vi "Dashboard Main.vi"() -> ()   [LabVIEW 2013]
uses:
  <vilib>/event_ctls.llb/eventvkey.ctl
  <vilib>/Rock Robotics/WPI/Dashboard/WPI_DashboardLogging Global.vi
  <vilib>/Utility/config.llb/Write Key (String).vi
  <vilib>/Utility/config.llb/Write Key (I32).vi
  <vilib>/Utility/config.llb/NI_LVConfig.lvlib
panel:
  out "Camera Image":T1(plugin-control)
  out "LED 1":bool
  out "Image Message":string="Timeout in Camera Communications"
  in  "Rec Mode":enum32{"Stop", "Record", "Playback"}(radio)
  in  "Dashboard Tab":T2(tab)
  out "Shooter":bool
  in  "Camera Settings":T3={"Frame Rate"=30, "Compression"=30, "Size"=1} {"Frame Rate" scale=1.0..30.0; "Size" items=["640x480", "320x240", "160x120"]}
  out "MotorSliders R":cluster{"MotorSlide1":dbl, "MotorSlide2":dbl} {"MotorSlide2" scale=-1.0..1.0 scale format="%#_2e"; "MotorSlide1" scale=-1.0..1.0 scale format="%#_2e"}
  out "MotorChart R":cluster{"Numeric":dbl, "Numeric":dbl}(graph)
  out "MotorSliders L":T4 {"MotorSlide4 2" scale=0.0..14.0 scale format="%#_2e"; "MotorSlide2" scale=-1.0..1.0 scale format="%#_2e"; "MotorSlide1" scale=-1.0..1.0 scale format="%#_2e"}
  out "MotorChart L":T5(graph)
  out "JS1 Z":dbl(slide) scale=-1.0..1.0 scale format="%#_2e"
  out "Joystick 1":cluster{"X":dbl, "Y":dbl}[](graph)
  out "JS Buttons 1":T6
  out "JS2 Z":dbl(slide) scale=-1.0..1.0 scale format="%#_2e"
  out "Joystick 2":cluster{"X":dbl, "Y":dbl}[](graph)
  out "JS Buttons 2":T6
  out "Mode":T7(ring)=enum."Auto Disabled"
  out "Camera IP":string
  in  "DB Camera Config":bool
  out "fps":dbl format="%#.1g"
  out "Mbps":dbl format="%#.1g"
  out "Mbps 2":bool
  out "You're\nGood\nHomie":bool
  out "Distance Meter":dbl(knob) scale=36.0..60.0
  in  "Slider 1":dbl(slide) scale=0.0..100.0
  in  "Checkbox 2":bool
  in  "Checkbox 1":bool
  in  "Test Slider":dbl(slide) scale=0.0..100.0 scale format="%#_3g"
  in  "On/Off":bool caption="Solenoid"
  in  "Test Name":u16(ring) items=["Select the test to run...", "Example Test", "-------------------------------", "List of tests is built in robot code.", "Replace with your own automated tests."]
  in  "Test Tree":string(tree)
  in  "Motor":cluster{"Value":dbl, "Enable":bool} {"Value" scale=-1.0..1.0 scale format="%#_3g"}
  out "Progress":T8 {"Test Progress" scale=0.0..100.0}
  in  "Rev/Fwd":cluster{"Forward":bool, "Reverse":bool}
  in  "Test Ring":u16(ring) items=["Auto", "Fixed indoor", "Fixed outdoor 1", "Fixed outdoor 2", "Fixed fluorescent 1", "Fixed fluorescent 2", "Hold current"]
  in  "Listbox":i32(listbox)
  out "Tree":string(tree)
  in  "Enable":bool
  # "Left"
  # "Front"
  # "Right"
  # "Battery"
  # "Customize by placing controls and indicators here and name to\nmatch Dashboard Variables on robot."
  # "This tab is a great place for autonomous settings and validation.\nCustomize by placing controls and indicators here and name to\nmatch Dashboard Variables on robot."
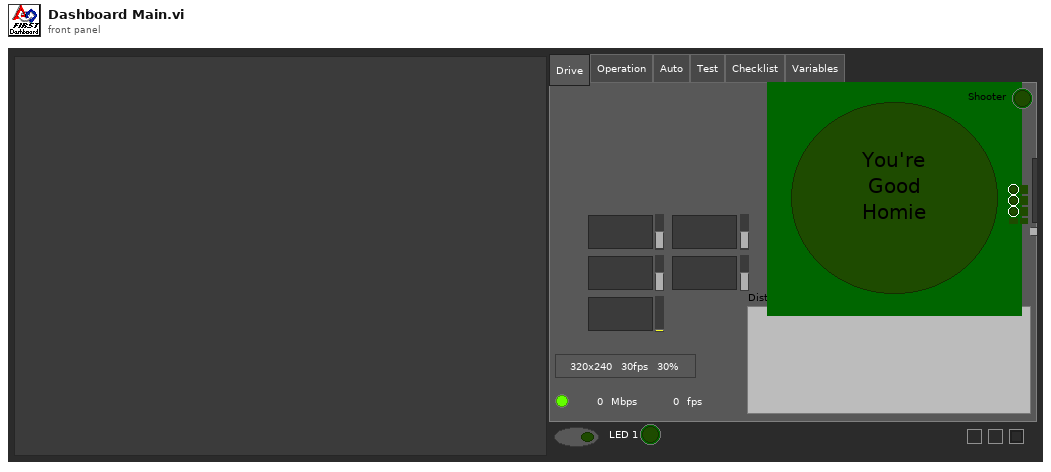
[diagram p1: front panel]
types:
  T1 = typedef "IMAQ Image.ctl" = refnum<image>
  T2 = enum32{"Drive", "Operation", "Auto", "Test", "Checklist", "Variables"}
  T3 = cluster{"Frame Rate":i32, "Compression":i32, "Size":u16}
  T4 = cluster{"MotorSlide1":dbl, "MotorSlide2":dbl, "MotorSlide4 2":dbl}
  T5 = cluster{"Numeric":dbl, "Numeric":dbl, "Battery":sgl}
  T6 = cluster{bool, bool, bool, bool, bool, bool, bool, bool, bool, bool, bool, bool}
  T7 = enum8{"Tele-Op Disabled", "Tele-Op Enabled", "Auto Disabled", "Auto Enabled", "Test Disabled", "Test Enabled", ""}
  T8 = cluster{"Test Progress":u8, "Test Progress Text":string}
  T9 = typedef "Image Type" = u32
  T10 = cluster{"X":bool, "A":bool, "B":bool, "Y":bool, "LB":bool, "RB":bool, "LT":bool, "RT":bool, "Back":bool, "Start":bool, "LC":bool, "RC":bool}
  T11 = cluster{"Pos. X":i32, "Pos. Y":i32, "Radius":i32, "Core Area":i32}[]
  T12 = cluster{"Pos. X":i32, "Pos. Y":i32, "Radius":i32, "Core Area":i32}
  T13 = typedef "NI_LVConfig.lvlib/Config Data RefNum.ctl" = refnum<k1>
  T14 = cluster{"Digital Inputs":bool[], "Digital Outputs":bool[]}
  T15 = cluster{"Competition mode":bool, "Robot Link":bool, "Autonomous":bool, "Enabled":bool, "E-Stop":bool, "Simulated":bool, "TestMode":bool, "Docked Window":bool}
  T16 = cluster{"Boolean Array[0]":bool, "Boolean Array[1]":bool, "Boolean Array[2]":bool, "Boolean Array[3]":bool, "Boolean Array[4]":bool, "Boolean Array[5]":bool, "Boolean Array[6]":bool, "Boolean Array[7]":bool, "Boolean Array[8]":bool, "Boolean Array[9]":bool, "Boolean Array[10]":bool, "Boolean Array[11]":bool}
  T17 = typedef "eventvkey.ctl" = enum16{"ASCII", "Enter", "Return", "Shift", "Ctrl", "Alt", "Cmd", "Opt", "Caps", "NumLock", "Clear", "Break", "Up", "Down", "Left", "Right", "Insert", "Delete", "Home", "End", "PageUp", "PageDown", "Escape", "Help", "Pause", "ScrollLock", "F1", "F2", "F3", "F4", "F5", "F6", "F7", "F8", "F9", "F10", "F11", "F12", "F13", "F14", "F15", "F16", "F17", "F18", "F19", "F20", "F21", "F22", "F23", "F24", "Play", "VolumeUp", "VolumeDown", "Mute", "Two Byte Char"}
  T18 = cluster{"Image Size":bool, "Image Type":bool, "Pixel Value":bool, "ROI Information":bool, "Zoom Factor":bool}
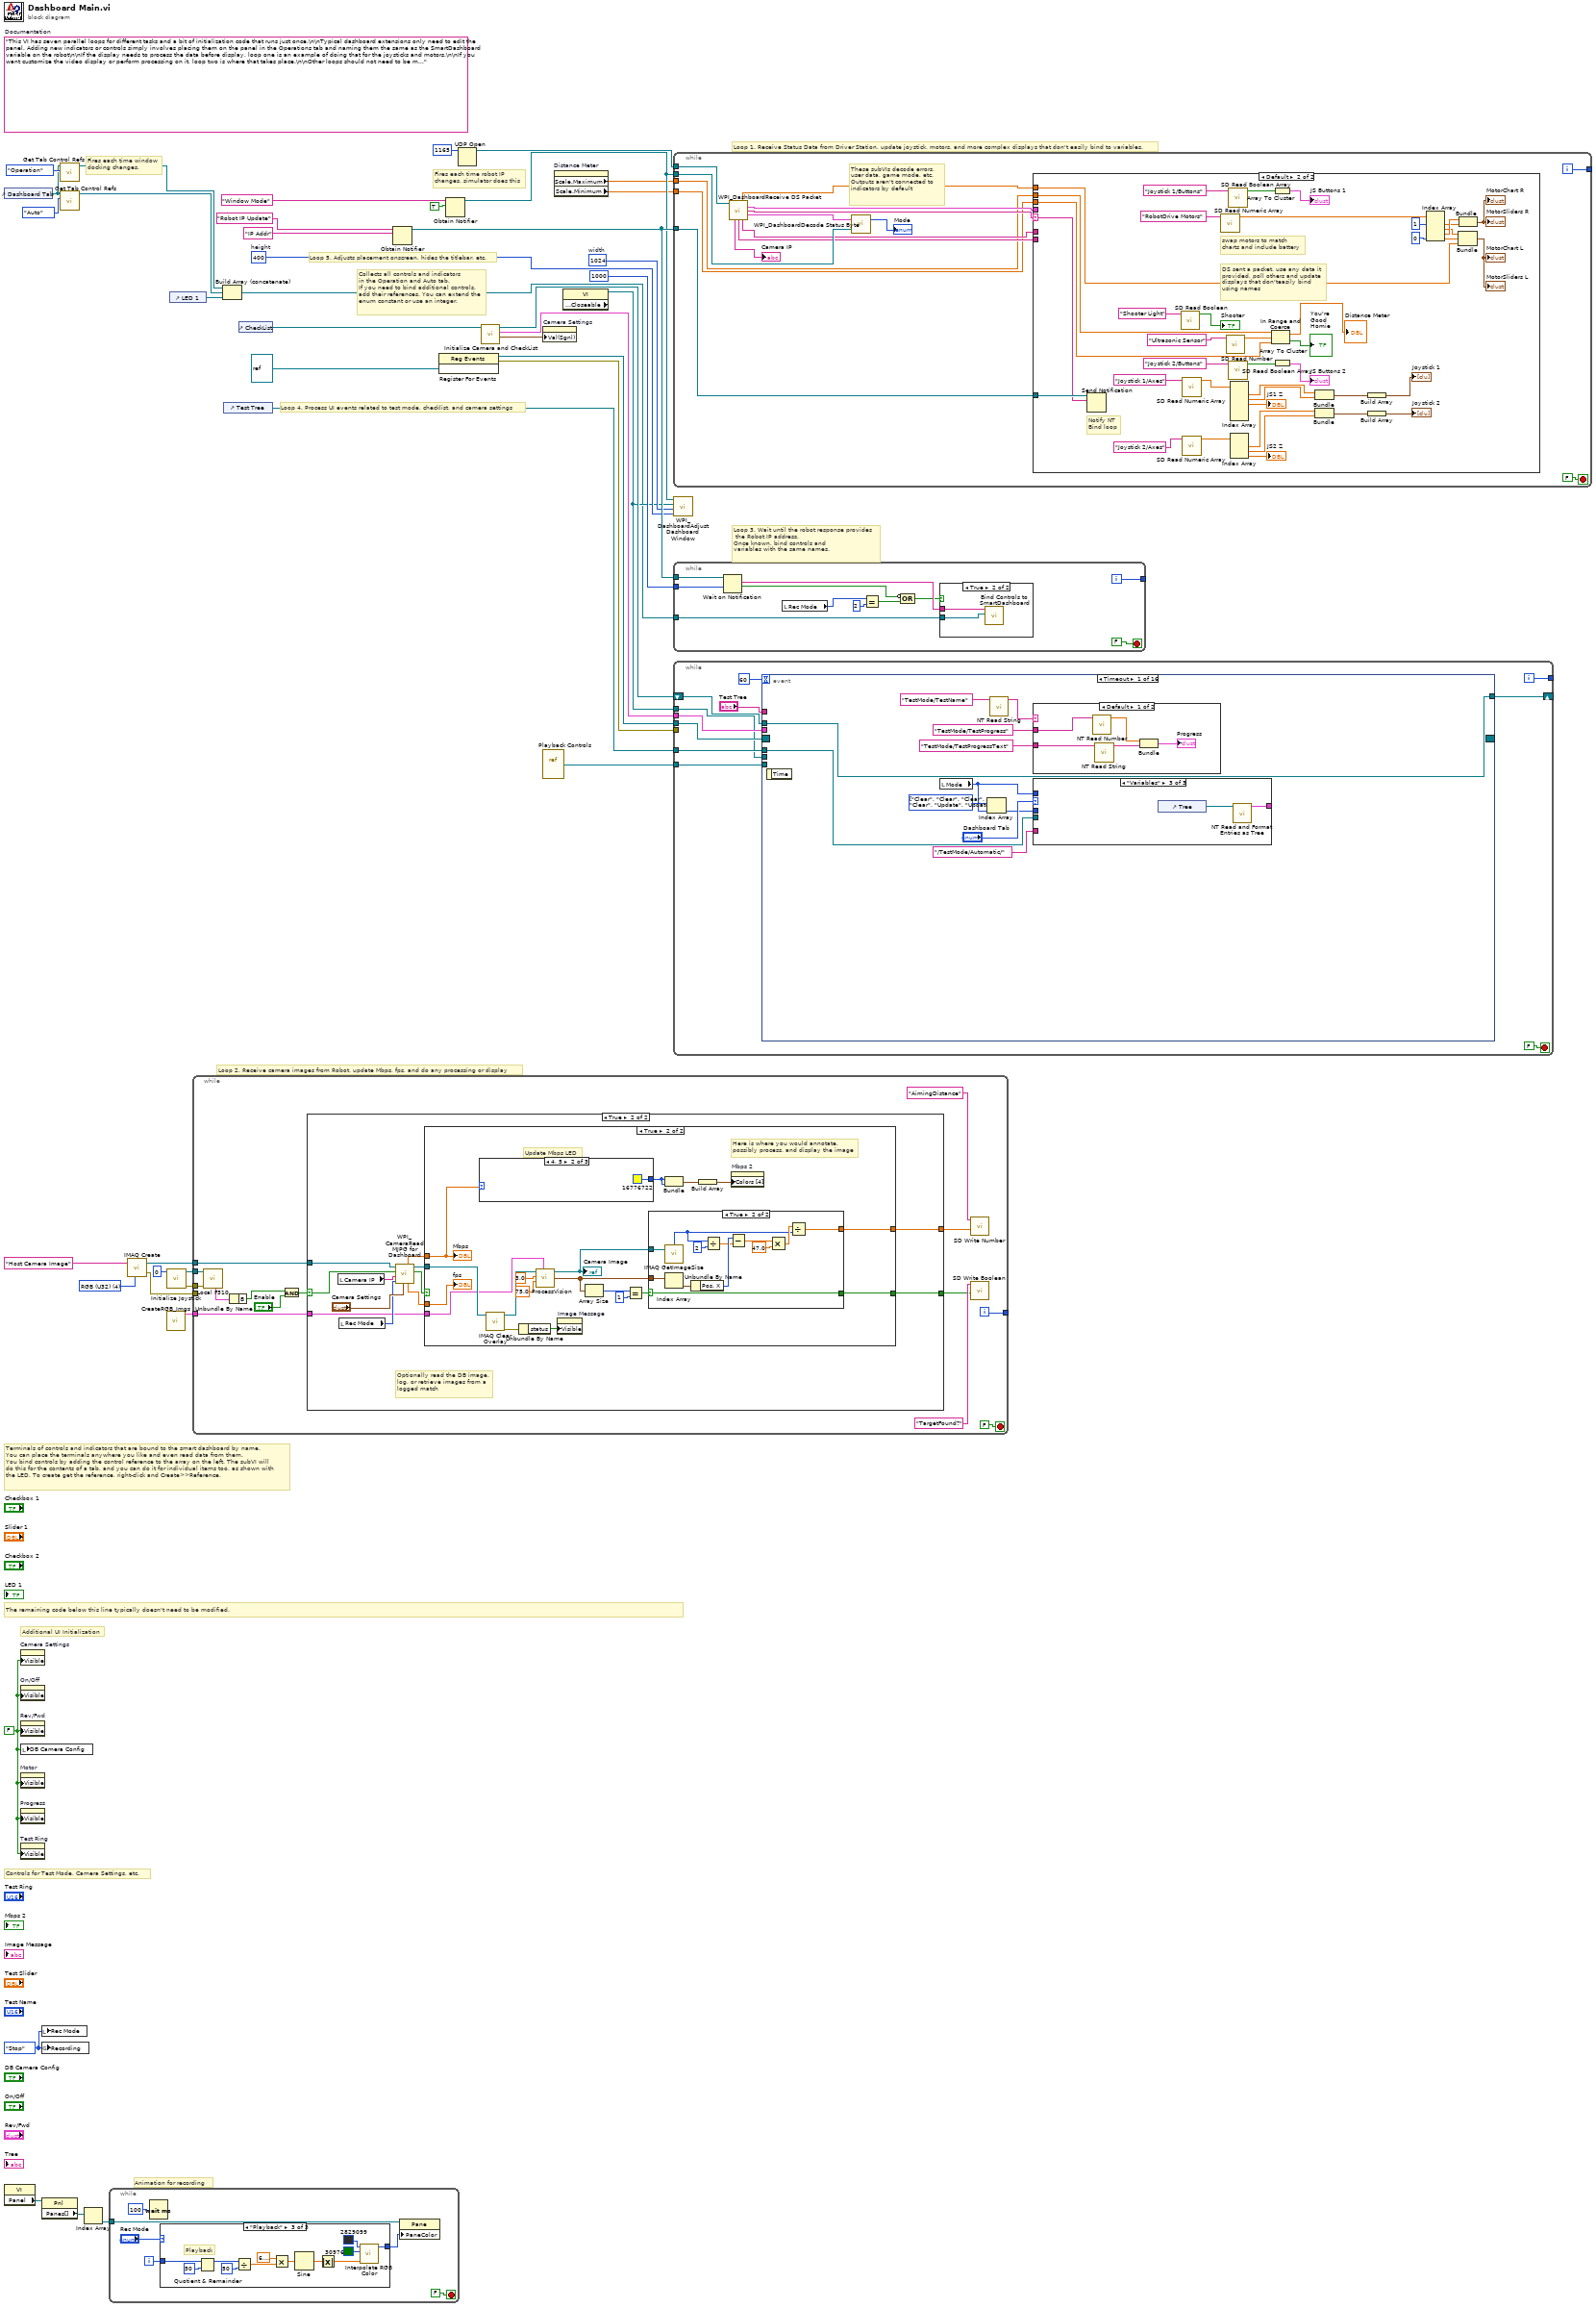
[diagram p0: block diagram]
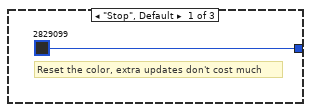
[diagram p2: hidden frame]
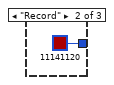
[diagram p3: hidden frame]
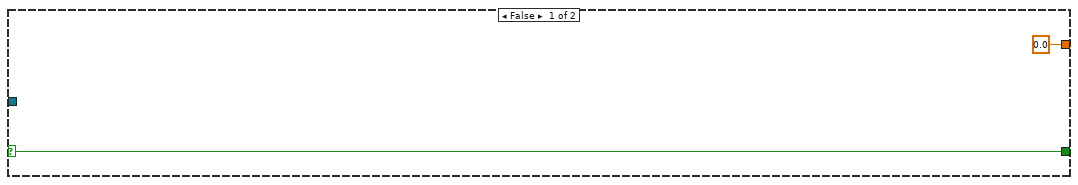
[diagram p5: hidden frame]
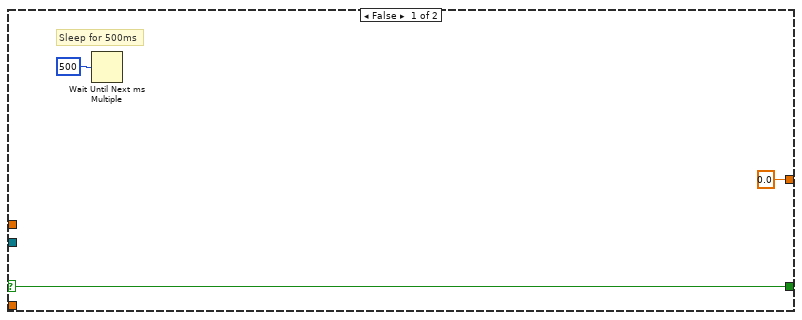
[diagram p6: hidden frame]
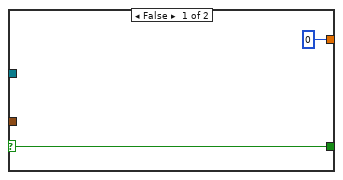
[diagram p7: hidden frame]
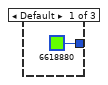
[diagram p8: hidden frame]
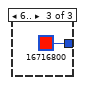
[diagram p9: hidden frame]
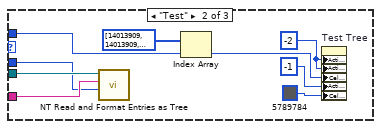
[diagram p11: hidden frame]
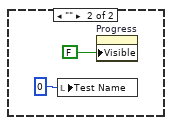
[diagram p12: hidden frame]
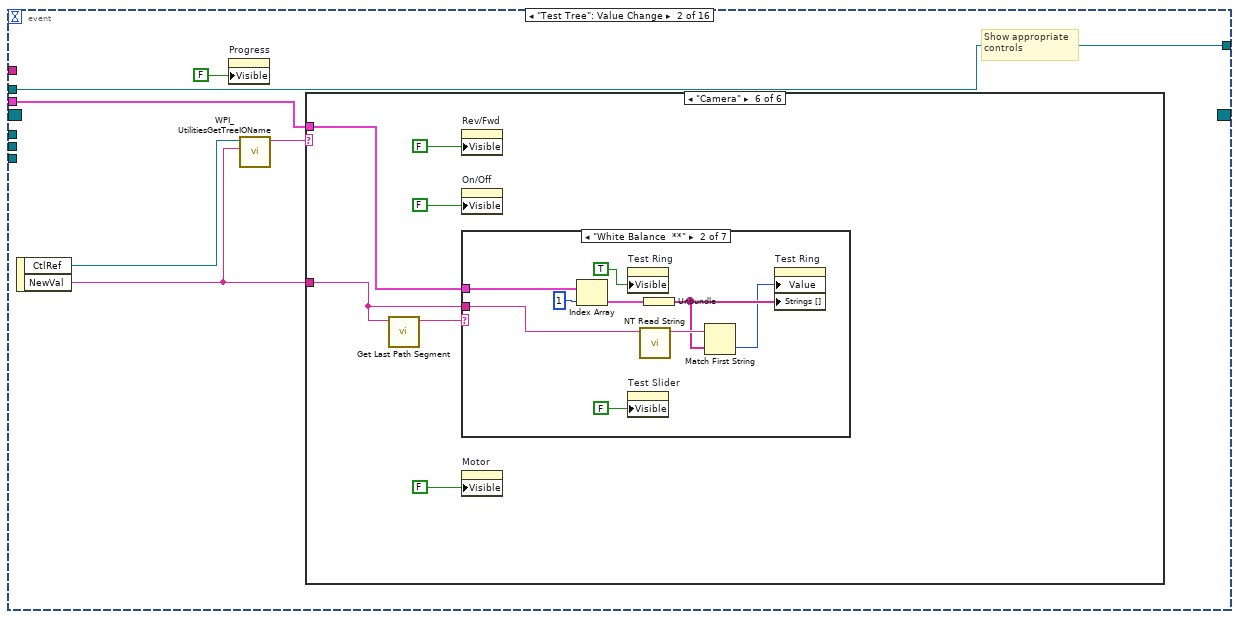
[diagram p13: hidden frame]
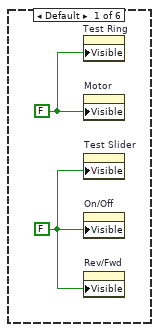
[diagram p14: hidden frame]
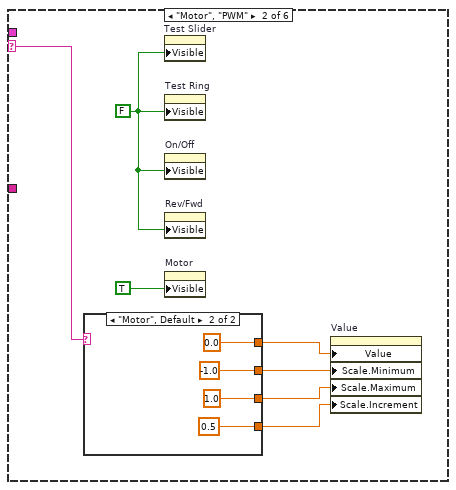
[diagram p15: hidden frame]
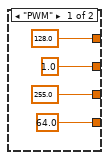
[diagram p16: hidden frame]
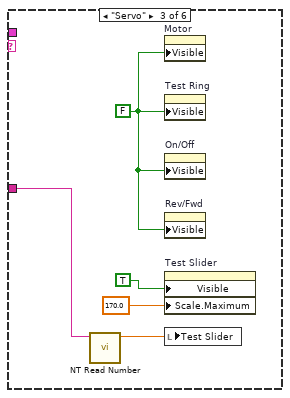
[diagram p17: hidden frame]
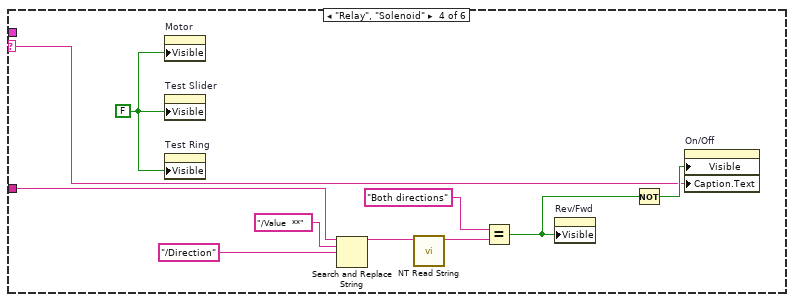
[diagram p18: hidden frame]
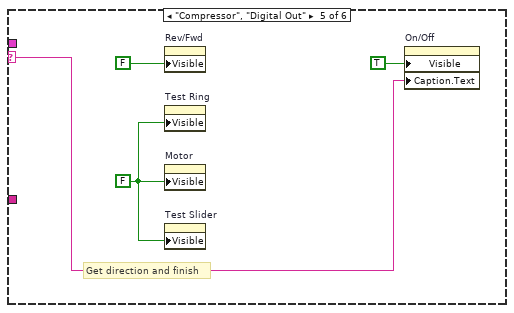
[diagram p19: hidden frame]
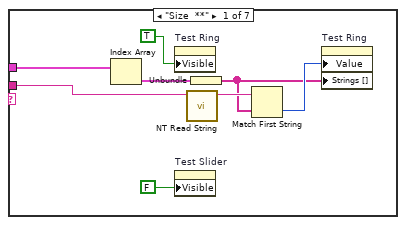
[diagram p20: hidden frame]
diagram:
  w14 = enum32{"Stop", "Record", "Playback"}."Stop" ("Rec Mode")
  w17 = 400  # height
  w18 = 1024  # width
  w31 = FALSE ("Visible")
  (unwired) "This VI has seven parallel loops for different tasks and a bit of initialization code that runs just once.\n\nTypical dashboard extensions only need to edit the panel. Adding new indicators or controls simply involves placing them on the panel in the Operations tab and naming them the same as the SmartDashboard variable on the robot\n\nIf the display needs to process the data before display, loop one is an example of doing that for the joysticks and motors.\n\nIf you want customize the video display or perform processing on it, loop two is where that takes place.\n\nOther loops should not need to be modified. They are pretty standard, and document the task they perform."  # Documentation
  w41 = T9 4 items=["Grayscale (U8)", "Grayscale (I16)", "Grayscale (SGL)", "Complex (CSG)", "RGB (U32)", "HSL (U32)", "RGB (U64)"] ("Image Type")
  # "Controls for Test Mode, Camera Settings, etc."
  # "Additional UI Initialization"
  # "Animation for recording"
  # "Fires each time robot IP\nchanges, simulator does this"
  # "Fires each time window\ndocking changes."
  # "Collects all controls and indicators\nin the Operation and Auto tab.\nIf you need to bind additional controls,\nadd their references. You can extend the\nenum constant or use an integer."
  # "The remaining code below this line typically doesn't need to be modified."
  # "Loop 4. Process UI events related to test mode, checklist, and camera settings"
  # "Terminals of controls and indicators that are bound to the smart dashboard by name.\nYou can place the terminals anywhere you like and even read data from them.\nYou bind controls by adding the control reference to the array on the left. The subVI will\ndo this for the contents of a tab, and you can do it for individual items too, as shown with\nthe LED. To create get the reference, right-click and Create>>Reference."
  # "Loop 3. Wait until the robot response provides\n the Robot IP address.\nOnce known, bind controls and\nvariables with the same names."
  # "Loop 5. Adjusts placement onscreen, hides the titlebar, etc."
  # "Loop 1. Receive Status Data from Driver Station, update joystick, motors, and more complex displays that don't easily bind to variables."
  # "Loop 2. Receive camera images from Robot, update Mbps, fps, and do any processing or display"
  n1 = control-ref of="Dashboard Tab"() -> (w12:refnum<vi>)
  n2 = property class="VI"() -> ("Panel"=w25:refnum<vi>)  [unwired: 2 in, 2 out]
  n3 = property on="Camera Settings" class="Clust (strict)"("Visible"=w31) -> ()  [unwired: 2 in, 2 out]
  n4 = property on="On/Off" class="Bool (strict)"("Visible"=w31) -> ()  [unwired: 2 in, 2 out]
  n5 = property on="Rev/Fwd" class="Clust (strict)"("Visible"=w31) -> ()  [unwired: 2 in, 2 out]
  n6 = local write "DB Camera Config"(w31) -> ()
  n7 = property on="Motor" class="Clust (strict)"("Visible"=w31) -> ()  [unwired: 2 in, 2 out]
  n8 = property on="Progress" class="Clust (strict)"("Visible"=w31) -> ()  [unwired: 2 in, 2 out]
  n9 = property on="Test Ring" class="Ring (strict)"("Visible"=w31) -> ()  [unwired: 2 in, 2 out]
  n10 = local write "Rec Mode"(w14) -> ()
  n11 = global write "WPI_DashboardLogging Global.vi" "Recording"(w14) -> ()
  n12 = property class="Pnl"(reference=w25) -> ("Panes[]"=w26:refnum<vi>[])  [unwired: 1 in, 2 out]
  n13 = call <vilib>:"Get Tab Control Refs.vi"("Page Index"=T2."Operation" ("Dashboard Tab"), "TabControl in"=w12) -> ("ControlsOnPage"=w10:refnum<vi>[])  [unwired: 9 in]
  n14 = call <vilib>:"Get Tab Control Refs.vi"("Page Index"=T2."Auto" ("Dashboard Tab"), "TabControl in"=w12) -> ("ControlsOnPage"=w11:refnum<vi>[])  [unwired: 9 in]
  n15 = Index Array(array=w26) -> (element=w24:refnum<vi>)  [unwired: 1 in]
  n16 = while {
    tunnel: w24 -> [w45]
    i -> [w48]
    stop <- FALSE stop-if-true
    n17 = Wait (ms)(milliseconds to wait=u32 100) -> ()  [unwired: 1 out]
    n18 = case shown="\"Playback\"" "Rec Mode" {
      tunnel: w48 -> [_ _ w63]
      tunnel: [u32 2829099 ("Base Color") u32 11141120 ("Target Color") w52] -> w44
      frame "Stop", Default {
        # "Reset the color, extra updates don't cost much"
      }
      frame "Record" {
      }
      frame "Playback" {
        # "Playback"
        n19 = Quotient & Remainder(x=w63, y=u32 50 ("milliseconds to wait")) -> (x-y*floor(x/y)=w59:u32)  [unwired: 1 out]
        n20 = Divide(x=w59, y=u32 50 ("milliseconds to wait")) -> (x/y=w56:dbl)
        n21 = Multiply(x=6.283185307179586, y=w56) -> (x*y=w61:dbl)
        n22 = Sine(x=w61) -> (sin(x)=w60:dbl)
        n23 = Absolute Value(x=w60) -> (abs(x)=w53:dbl)
        n24 = call "Interpolate RGB Color.vi"("Proportion"=w53, "Target Color"=u32 30976, "Base Color"=u32 2829099) -> ("Result Color"=w52:u32)  [unwired: 8 in]
      }
    }
    n25 = property class="Pane"(reference=w45, "PaneColor"=w44) -> ()  [unwired: 1 in, 2 out]
  }
  n26 = call "IMAQ Create"("Image Name"="Host Camera Image", "Image Type"=w41) -> ("New Image"=w39:T1, "error out"=w38:errorcluster)  [unwired: 2 in, 1 out]
  n27 = call "CreateRGB_Imgs.vi"() -> ("RGB Cluster"=w4:cluster{"Red":T1, "Green":T1, "Blue":T1})  [unwired: 3 out]
  n28 = call <vilib>:"Initialize Joystick.vi"("device index"=0) -> ("error out"=w2:errorcluster, "device ID"=w1:refnum<k1>)  [unwired: 9 in]
  n29 = control-ref of="LED 1"() -> (w7:refnum<vi>)
  n30 = while {
    tunnel: w39 -> [w75]
    tunnel: w38 -> [_]
    tunnel: [w76] -> _
    tunnel: w4 -> [w73]
    tunnel: w2 -> [w72]
    tunnel: w1 -> [w71]
    i -> [w76]
    stop <- FALSE stop-if-true
    n31 = call "Local F310.vi"("error in (no error)"=w72, "device ID"=w71) -> ("Buttons"=w70:T10)  [unwired: 4 in, 5 out]
    n32 = Unbundle By Name(w70) -> ("B"=w69:bool)
    n33 = And(x=w69, y="Enable") -> (x .and. y?=w68:bool)
    n34 = case shown="True" w68 {
      selector: w68 -> [w79 w80]
      tunnel: w75 -> [_ w91]
      tunnel: w73 -> [_ w83]
      tunnel: [0.0 ("Pos. X") w82] -> w65
      tunnel: [w79 w81] -> w64
      frame False {
      }
      frame True {
        # "Optionally read the DB image,\nlog, or retrieve images from a\nlogged match"
        n35 = local read "Camera IP"() -> (w85:string)
        n36 = local read "Rec Mode"() -> (w84:enum32{"Stop", "Record", "Playback"})
        n37 = call <vilib>:"WPI_CameraRead MJPG for Dashboard.vi"("Camera Settings"="Camera Settings", "Rec Mode"=w84, "Camera IP"=w85, "Enable"=w80, "Refnum in"=w91) -> ("Active"=w89:bool, "Refnum out"=w90:T1, "FPS"=w88:dbl, "Bandwidth (Mbps)"=w87:dbl)  [unwired: 3 in]
        n38 = case shown="True" w89 {
          selector: w89 -> [w93 _]
          tunnel: w90 -> [_ w108]
          tunnel: w87 -> [_ w107]
          tunnel: w88 -> [_ w106]
          tunnel: w83 -> [_ w98]
          tunnel: [0.0 ("Pos. X") w96] -> w82
          tunnel: [w93 w95] -> w81
          frame False {
            # "Sleep for 500ms"
            n39 = Wait Until Next ms Multiple(millisecond multiple=u32 500) -> ()  [unwired: 1 out]
          }
          frame True {
            # "Here is where you would annotate,\npossibly process, and display the image"
            # "Update Mbps LED"
            n40 = case shown="4, 5" w107 {
              tunnel: [u32 6618880 ("Color Box") u32 16776722 ("Color Box") u32 16716800 ("Color Box")] -> w109
              frame Default {
              }
              frame 4, 5 {
              }
              frame 6.. {
              }
            }
            n41 = call "IMAQ Clear Overlay"("Image"=w108) -> ("error out"=w112:errorcluster, "Image Out"=w102:T1)  [unwired: 2 in, 7 out]
            n42 = Unbundle By Name(w112) -> ("status"=w113:bool)
            n43 = call "ProcessVision.vi"("Image Src"=w102, "Min Radius"=sgl 3.0, "Max Radius"=sgl 75.0, "RGB Cluster"=w98) -> ("Image Out"=w97:T1, "Circles Data"=w99:T11)  [unwired: 1 in, 1 out]
            "Camera Image" <- w97
            n44 = property on="Image Message" class="Str"("Visible"=w113) -> ()  [unwired: 2 in, 2 out]
            n45 = Array Size(array=w99) -> (size(s)=w105:i32)
            n46 = Equal?(x=w105, y=1) -> (x = y?=w103:bool)
            n47 = case shown="True" w103 {
              selector: w103 -> [w114 w127]
              tunnel: [0 ("Pos. X") w116] -> w96
              tunnel: [w114 w127] -> w95
              tunnel: w99 -> [_ w126]
              tunnel: w97 -> [_ w124]
              frame False {
              }
              frame True {
                n48 = call "IMAQ GetImageSize"("Image"=w124) -> ("X Resolution"=w117:i32)  [unwired: 3 in, 2 out]
                n49 = Index Array(array=w126) -> (element=w125:T12)  [unwired: 1 in]
                n50 = Unbundle By Name(w125) -> ("Pos. X"=w122:i32)
                n51 = Divide(x=w117, y=2) -> (x/y=w121:dbl)
                n52 = Subtract(x=w122, y=w121) -> (x-y=w120:dbl)
                n53 = Multiply(x=w120, y=47.0) -> (x*y=w118:dbl)
                n54 = Divide(x=w118, y=w117) -> (x/y=w116:dbl)
              }
            }
            n55 = Bundle("Color Box"=w109, "Color Box"=w109) -> (w111:cluster{"Color Box":u32, "Color Box":u32})  [unwired: 1 out]
            n56 = Build Array(w111) -> (w110:cluster{"Color Box":u32, "Color Box":u32}[])
            n57 = property on="Mbps 2" class="Bool (strict)"("Colors [4]"=w110) -> ()  [unwired: 2 in, 2 out]
            "Mbps" <- w107
            "fps" <- w106
          }
        }
      }
    }
    n58 = call <vilib>:"SD Write Number.vi"("Numeric"=w65, "Name"="AimingDistance") -> ()  [unwired: 8 in, 2 out]
    n59 = call <vilib>:"SD Write Boolean.vi"("Boolean"=w64, "Name"="TargetFound?") -> ()  [unwired: 8 in, 2 out]
  }
  n60 = Build Array (concatenate)(w10, w11, w7) -> (w9:refnum<vi>[])
  n61 = control-ref of="Test Tree"() -> (w27:refnum<vi>)
  n62 = control-ref of="CheckList"() -> (w15:refnum<vi>)
  n63 = Obtain Notifier(name (unnamed)="Robot IP Update", notification data type="IP Addr" ("name (unnamed)")) -> (notifier out=w35:refnum<notifier>)  [unwired: 2 in, 2 out]
  n64 = register-events(refnum<vi> refnum) -> (reference out=w22:refnum<event-registration>, error out=w21:errorcluster)  [unwired: 2 in]
  n65 = Obtain Notifier(name (unnamed)="Window Mode", notification data type=TRUE) -> (notifier out=w16:refnum<notifier>)  [unwired: 2 in, 2 out]
  n66 = UDP Open(11:u16 1165 ("port")) -> (port=w42:refnum<k16>)  [unwired: 2 in, 4 out]
  n67 = call "Initialize Camera and CheckList.vi"("ListBox in"=w15) -> ("Cluster"=w29:cluster{"value":i32, "value":i32, "index":i32}, "Array"=w30:cluster{string[]}[], "File Refnum"=w28:T13)  [unwired: 8 in]
  n68 = property on="Camera Settings" class="Clust (strict)"("Val(Sgnl)"=w29) -> ()  [unwired: 2 in, 2 out]
  n69 = vi-ref "Playback Controls.vi"() -> (w23:refnum<vi>)
  n70 = property on="Distance Meter" class="Knob (strict)"() -> ("Scale.Maximum"=w6:dbl, "Scale.Minimum"=w5:dbl)  [unwired: 2 in, 2 out]
  n71 = property class="VI" props=["Front Panel.Closeable"]() -> (reference out=w13:refnum<vi>)  [unwired: 2 in, 2 out]
  n72 = while {
    tunnel: w42 -> [w143]
    tunnel: w35 -> [w138]
    tunnel: w16 -> [w142]
    tunnel: [w139] -> _
    tunnel: w6 -> [w132]
    tunnel: w5 -> [w131]
    i -> [w139]
    stop <- FALSE stop-if-true
    # "These subVIs decode errors, user data, game mode, etc.\nOutputs aren't connected to indicators by default"
    n73 = call <vilib>:"WPI_DashboardReceive DS Packet.vi"("Recv Socket"=w143) -> ("Battery"=w133:sgl, "Driver Station"=w134:T14, "Robot IP Address"=w137:string, "Status"=w144:T15, "Camera IP Address"=→"Camera IP":string, "Low Priority User Data"=w136:string, "High Priority User Data"=w135:string)  [unwired: 1 in, 7 out]
    n74 = call <vilib>:"WPI_DashboardDecode Status Byte.vi"("Window Mode Notifier"=w142, "Status"=w144) -> ("Mode"=→"Mode":T7)  [unwired: 1 out]
    n75 = case shown="Default" w137 {
      selector: w137 -> [_ w164]
      tunnel: w138 -> [_ w165]
      tunnel: w136 -> [_ _]
      tunnel: w135 -> [_ _]
      tunnel: w134 -> [_ _]
      tunnel: w133 -> [_ w163]
      tunnel: w132 -> [_ w149]
      tunnel: w131 -> [_ w150]
      frame "0.0.0.0" {
        # "DS not sending packets, or no robot exists yet.\nDon't poll the variables"
      }
      frame Default {
        # "Notify NT\nBind loop"
        # "DS sent a packet. use any data it\nprovided, poll others and update\ndisplays that don'teasily bind\nusing names"
        # "swap motors to match\ncharts and include battery"
        n76 = Send Notification(notification=w164, notifier=w165) -> ()  [unwired: 1 in, 2 out]
        n77 = call <vilib>:"SD Read Boolean.vi"("Name"="Shooter Light") -> ("Boolean"=→"Shooter":bool)  [unwired: 8 in, 2 out]
        n78 = call <vilib>:"SD Read Numeric Array.vi"("Name"="Joystick 1/Axes") -> ("Numeric Array"=w181:dbl[])  [unwired: 8 in, 2 out]
        n79 = call <vilib>:"SD Read Numeric Array.vi"("Name"="Joystick 2/Axes") -> ("Numeric Array"=w175:dbl[])  [unwired: 8 in, 2 out]
        n80 = call <vilib>:"SD Read Numeric Array.vi"("Name"="RobotDrive Motors") -> ("Numeric Array"=w162:dbl[])  [unwired: 8 in, 2 out]
        n81 = call <vilib>:"SD Read Number.vi"("Name"="Ultrasonic Sensor") -> ("Numeric"=w151:dbl)  [unwired: 8 in, 2 out]
        n82 = call <vilib>:"SD Read Boolean Array.vi"("Name"="Joystick 1/Buttons") -> ("Boolean Array"=w183:bool[])  [unwired: 8 in, 2 out]
        n83 = call <vilib>:"SD Read Boolean Array.vi"("Name"="Joystick 2/Buttons") -> ("Boolean Array"=w174:bool[])  [unwired: 8 in, 2 out]
        n84 = Index Array(array=w181) -> (element #1=w178:dbl, element #2=w179:dbl, element #3=→"JS1 Z":dbl)  [unwired: 6 in, 3 out]
        n85 = Index Array(array=w175) -> (element #1=w170:dbl, element #2=w169:dbl, element #3=→"JS2 Z":dbl)  [unwired: 3 in]
        n86 = In Range and Coerce(upper limit=w149, x=w151, lower limit=w150) -> (coerced(x)=→"Distance Meter":dbl, In Range?=→"You're\nGood\nHomie":bool)
        n87 = Array To Cluster(array=w183) -> (cluster=→"JS Buttons 1":T16)
        n88 = Array To Cluster(array=w174) -> (cluster=→"JS Buttons 2":T16)
        n89 = Bundle("Numeric"=w178, "Numeric"=w179) -> (w177:cluster{"Numeric":dbl, "Numeric":dbl})  [unwired: 1 in]
        n90 = Bundle("Numeric"=w170, "Numeric"=w169) -> (w171:cluster{"Numeric":dbl, "Numeric":dbl})  [unwired: 1 in]
        n91 = Build Array(w177) -> (→"Joystick 1":cluster{"Numeric":dbl, "Numeric":dbl}[])
        n92 = Build Array(w171) -> (→"Joystick 2":cluster{"Numeric":dbl, "Numeric":dbl}[])
        n93 = Index Array(array=w162, index #1=1, index #4=0) -> (element #1=w158:dbl, element #2=w157:dbl, element #3=w159:dbl, element #4=w154:dbl)  [unwired: 2 in]
        n94 = Bundle("Numeric"=w157, "Numeric"=w154, "Battery"=w163) -> (→"MotorChart L" →"MotorSliders L":T5)  [unwired: 1 in]
        n95 = Bundle("Numeric"=w159, "Numeric"=w158) -> (→"MotorChart R" →"MotorSliders R":cluster{"Numeric":dbl, "Numeric":dbl})  [unwired: 1 in]
      }
    }
  }
  n96 = call <vilib>:"WPI_DashboardAdjust Dashboard Window.vi"("height"=w17, "width"=w18, "reference in"=w13, "Notifier in"=w16) -> ()  [unwired: 8 in]
  n97 = while {
    tunnel: w9 -> [w197]
    tunnel: w35 -> [w195]
    tunnel: [w193] -> _
    tunnel: u32 1000 ("milliseconds to wait") -> [w192]
    i -> [w193]
    stop <- FALSE stop-if-true
    n98 = Wait on Notification(notifier=w195, timeout in ms (-1)=w192) -> (notification=w194:string, timed out?=w190:bool)  [unwired: 2 in, 2 out]
    n99 = local read "Rec Mode"() -> (w188:enum32{"Stop", "Record", "Playback"})
    n100 = Equal?(x=w188, y=u16 2 ("Rec Mode")) -> (x = y?=w189:bool)
    n101 = Compound Arithmetic op=OR(invert w190, w189) -> (w191:bool)
    n102 = case shown="True" w191 {
      tunnel: w197 -> [_ w199]
      tunnel: w194 -> [_ w198]
      frame False {
      }
      frame True {
        n103 = call <vilib>:"Bind Controls to SmartDashboard.vi"("Bound Control Refs"=w199, "Server IP Address"=w198) -> ()  [unwired: 10 in]
      }
    }
  }
  n104 = while {
    tunnel: w30 -> [w207]
    shift-right: [w206] -> _
    shift-left: w28 -> [w205]
    tunnel: [w204] -> _
    tunnel: w27 -> [w203]
    tunnel: w23 -> [w202]
    tunnel: w22 -> [w201]
    tunnel: w21 -> [_]
    tunnel: w13 -> [w200]
    i -> [w204]
    stop <- FALSE stop-if-true
    n105 = event shown="[0] Timeout" {
      selector: w201 -> [_ _ _ _ _ _ _ _ _ _ _ _ _ _ _ _]
      dyn-events: [_ _ _ _ _ _ _ _ _ _ _ _ _ w443 _ _] -> _
      timeout: u32 60 ("milliseconds to wait") -> [_ _ _ _ _ _ _ _ _ _ _ _ _ _ _ _]
      tunnel: w203 -> [w217 _ _ _ _ _ _ _ _ _ _ _ _ _ _ _]
      tunnel: "Test Tree" -> [_ _ _ _ _ _ _ _ w414 w422 w424 w428 w436 _ _ _]
      tunnel: w207 -> [_ w241 _ _ _ _ w378 w408 _ _ _ _ _ _ _ _]
      tunnel: [w211 w240 w339 w344 w352 w364 w377 w401 w413 w420 w423 w427 w435 w445 w459 w460] -> w206
      tunnel: w205 -> [w211 w240 w339 w344 w352 w364 w376 w401 w413 w420 w423 w427 w435 w445 w459 w460]
      tunnel: w202 -> [_ _ _ _ _ _ _ _ _ _ _ _ _ w446 _ w463]
      tunnel: w200 -> [_ _ _ _ _ _ _ _ _ _ _ _ _ w441 _ _]
      event Timeout {
        w216 = enum16{"Update", "Clear"}[] [enum."Clear", enum."Clear", enum."Clear", enum."Clear", enum."Update", enum."Update", enum."Clear"] items=["Update", "Clear"]
        n106 = event-data() -> ()  [unwired: 1 in, 1 out]
        n107 = local read "Mode"() -> (w214:T7)
        n108 = Index Array(array=w216, index=w214) -> (element=w215:enum16{"Update", "Clear"})
        n109 = call <vilib>:"NT Read String.vi"("Name"="TestMode/TestName") -> ("String"=w220:string)  [unwired: 9 in, 1 out]
        n110 = case shown="Default" w220 {
          tunnel: "TestMode/TestProgress" ("Name") -> [w234 _]
          tunnel: "TestMode/TestProgressText" ("Name") -> [w233 _]
          frame Default {
            n111 = call <vilib>:"NT Read Number.vi"("Name"=w234) -> ("Numeric"=w235:dbl)  [unwired: 9 in, 1 out]
            n112 = call <vilib>:"NT Read String.vi"("Name"=w233) -> ("String"=w236:string)  [unwired: 9 in, 1 out]
            n113 = Bundle("Numeric"=w235, "String"=w236) -> (→"Progress":cluster{"Numeric":dbl, "String":string})  [unwired: 1 in]
          }
          frame "" {
            n114 = local write "Test Name"(u16 0) -> ()
            n115 = property on="Progress" class="Clust (strict)"("Visible"=FALSE) -> ()  [unwired: 2 in, 2 out]
          }
        }
        n116 = case shown="\"Variables\"" "Dashboard Tab" {
          tunnel: w217 -> [_ w230 _]
          tunnel: "/TestMode/Automatic/" ("Name Pattern") -> [_ w229 _]
          tunnel: w215 -> [_ w228 _]
          tunnel: w214 -> [_ w226 _]
          tunnel: [_ _ w232] -> _
          frame "Operation", Default {
          }
          frame "Test" {
            w225 = -2 ("Active Item:Row Number")
            n117 = call <vilib>:"NT Read and Format Entries as Tree.vi"("Operation"=w228, "Name Pattern"=w229, "Tree Refnum"=w230) -> ()  [unwired: 7 in, 2 out]
            n118 = Index Array(array=u32[] [14013909, 14013909, 14013909, 14013909, 14013909, 16777215, 14013909], index=w226) -> (element=w224:u32)
            n119 = property on="Test Tree" class="Tree (strict)"("Active Item Row Number"=w225, "ActiveColNum"=w225, "CellBG"=w224, "Active Item Row Number"=-1 ("Active Item:Row Number"), "CellBG"=u32 5789784 ("Color Box")) -> ()  [unwired: 2 in, 2 out]
          }
          frame "Variables" {
            n120 = control-ref of="Tree"() -> (w231:refnum<vi>)
            n121 = call <vilib>:"NT Read and Format Entries as Tree.vi"("Tree Refnum"=w231) -> ("Formatted Strings"=w232:cluster{"Name":string, "Value":string}[])  [unwired: 9 in, 1 out]
          }
        }
      }
      event "Test Tree": Value Change {
        # "Show appropriate\ncontrols"
        n122 = event-data() -> ("CtlRef"=w244:refnum<vi>, "NewVal"=w242:string)  [unwired: 1 in]
        n123 = property on="Progress" class="Clust (strict)"("Visible"=FALSE) -> ()  [unwired: 2 in, 2 out]
        n124 = call <vilib>:"WPI_UtilitiesGetTreeIOName.vi"("NewVal"=w242, "TreeControl in"=w244) -> ("I/O Name"=w245:string)  [unwired: 9 in]
        n125 = case shown="\"Camera\"" w245 {
          selector: w245 -> [_ w252 _ w270 w279 _]
          tunnel: w242 -> [_ _ w267 w269 _ w286]
          tunnel: w241 -> [_ _ _ _ _ w285]
          frame Default {
            w247 = FALSE ("Visible")
            w246 = FALSE ("Visible")
            n126 = property on="Test Ring" class="Ring (strict)"("Visible"=w246) -> ()  [unwired: 2 in, 2 out]
            n127 = property on="Motor" class="Clust (strict)"("Visible"=w246) -> ()  [unwired: 2 in, 2 out]
            n128 = property on="Test Slider" class="Slide (strict)"("Visible"=w247) -> ()  [unwired: 2 in, 2 out]
            n129 = property on="On/Off" class="Bool (strict)"("Visible"=w247) -> ()  [unwired: 2 in, 2 out]
            n130 = property on="Rev/Fwd" class="Clust (strict)"("Visible"=w247) -> ()  [unwired: 2 in, 2 out]
          }
          frame "Motor", "PWM" {
            w253 = FALSE ("Visible")
            n131 = case shown="\"Motor\", Default" w252 {
              tunnel: [1.0 ("Value") -1.0 ("Value")] -> w251
              tunnel: [255.0 ("Value") 1.0 ("Value")] -> w250
              tunnel: [128.0 ("Value") 0.0 ("Value")] -> w249
              tunnel: [64.0 ("Value") 0.5 ("Value")] -> w248
              frame "PWM" {
              }
              frame "Motor", Default {
              }
            }
            n132 = property on="Test Slider" class="Slide (strict)"("Visible"=w253) -> ()  [unwired: 2 in, 2 out]
            n133 = property on="Test Ring" class="Ring (strict)"("Visible"=w253) -> ()  [unwired: 2 in, 2 out]
            n134 = property on="On/Off" class="Bool (strict)"("Visible"=w253) -> ()  [unwired: 2 in, 2 out]
            n135 = property on="Rev/Fwd" class="Clust (strict)"("Visible"=w253) -> ()  [unwired: 2 in, 2 out]
            n136 = property on="Motor" class="Clust (strict)"("Visible"=TRUE) -> ()  [unwired: 2 in, 2 out]
            n137 = property on="Value" class="Slide (strict)"("Value"=w249, "Scale.Minimum"=w251, "Scale.Maximum"=w250, "Scale.Increment"=w248) -> ()  [unwired: 2 in, 2 out]
          }
          frame "Servo" {
            w265 = FALSE ("Visible")
            n138 = call <vilib>:"NT Read Number.vi"("Name"=w267) -> ("Numeric"=w266:dbl)  [unwired: 9 in, 1 out]
            n139 = property on="Motor" class="Clust (strict)"("Visible"=w265) -> ()  [unwired: 2 in, 2 out]
            n140 = property on="Test Ring" class="Ring (strict)"("Visible"=w265) -> ()  [unwired: 2 in, 2 out]
            n141 = property on="On/Off" class="Bool (strict)"("Visible"=w265) -> ()  [unwired: 2 in, 2 out]
            n142 = property on="Rev/Fwd" class="Clust (strict)"("Visible"=w265) -> ()  [unwired: 2 in, 2 out]
            n143 = property on="Test Slider" class="Slide (strict)"("Visible"=TRUE, "Scale.Maximum"=170.0 ("Scale.Range:Maximum")) -> ()  [unwired: 2 in, 2 out]
            n144 = local write "Test Slider"(w266) -> ()
          }
          frame "Relay", "Solenoid" {
            w268 = FALSE ("Visible")
            n145 = property on="Motor" class="Clust (strict)"("Visible"=w268) -> ()  [unwired: 2 in, 2 out]
            n146 = property on="Test Slider" class="Slide (strict)"("Visible"=w268) -> ()  [unwired: 2 in, 2 out]
            n147 = property on="Test Ring" class="Ring (strict)"("Visible"=w268) -> ()  [unwired: 2 in, 2 out]
            n148 = Search and Replace String(input string=w269, search string="/Value  **", replace string="/Direction") -> (result string=w275:string)  [unwired: 5 in, 3 out]
            n149 = call <vilib>:"NT Read String.vi"("Name"=w275) -> ("String"=w273:string)  [unwired: 9 in, 1 out]
            n150 = Equal?(x="Both directions", y=w273) -> (x = y?=w271:bool)
            n151 = property on="Rev/Fwd" class="Clust (strict)"("Visible"=w271) -> ()  [unwired: 2 in, 2 out]
            n152 = Not(x=w271) -> (.not. x?=w272:bool)
            n153 = property on="On/Off" class="Bool (strict)"("Visible"=w272, "Caption.Text"=w270) -> ()  [unwired: 2 in, 2 out]
          }
          frame "Compressor", "Digital Out" {
            w278 = FALSE ("Visible")
            # "Get direction and finish"
            n154 = property on="Rev/Fwd" class="Clust (strict)"("Visible"=FALSE) -> ()  [unwired: 2 in, 2 out]
            n155 = property on="Test Ring" class="Ring (strict)"("Visible"=w278) -> ()  [unwired: 2 in, 2 out]
            n156 = property on="Motor" class="Clust (strict)"("Visible"=w278) -> ()  [unwired: 2 in, 2 out]
            n157 = property on="Test Slider" class="Slide (strict)"("Visible"=w278) -> ()  [unwired: 2 in, 2 out]
            n158 = property on="On/Off" class="Bool (strict)"("Visible"=TRUE, "Caption.Text"=w279) -> ()  [unwired: 2 in, 2 out]
          }
          frame "Camera" {
            n159 = call <vilib>:"Get Last Path Segment.vi"("String in"=w286) -> ("String out"=w287:string)  [unwired: 10 in]
            n160 = property on="Rev/Fwd" class="Clust (strict)"("Visible"=FALSE) -> ()  [unwired: 2 in, 2 out]
            n161 = property on="On/Off" class="Bool (strict)"("Visible"=FALSE) -> ()  [unwired: 2 in, 2 out]
            n162 = case shown="\"White Balance  **\"" w287 {
              tunnel: w286 -> [w293 w302 w311 w320 w329 _ w335]
              tunnel: w285 -> [w291 w299 w308 w317 w326 _ _]
              frame "Size  **" {
                n163 = Index Array(array=w291) -> (element=w290:cluster{string[]})  [unwired: 1 in]
                n164 = property on="Test Ring" class="Ring (strict)"("Visible"=TRUE) -> ()  [unwired: 2 in, 2 out]
                n165 = property on="Test Slider" class="Slide (strict)"("Visible"=FALSE) -> ()  [unwired: 2 in, 2 out]
                n166 = call <vilib>:"NT Read String.vi"("Name"=w293) -> ("String"=w292:string)  [unwired: 9 in, 1 out]
                n167 = Unbundle(w290) -> (w288:string[])
                n168 = Match First String(2:w288, 3:w292) -> (0:w289:i32)  [unwired: 1 out]
                n169 = property on="Test Ring" class="Ring (strict)"("Value"=w289, "Strings []"=w288) -> ()  [unwired: 2 in, 2 out]
              }
              frame "White Balance  **" {
                n170 = Index Array(array=w299, index=1) -> (element=w300:cluster{string[]})
                n171 = property on="Test Ring" class="Ring (strict)"("Visible"=TRUE) -> ()  [unwired: 2 in, 2 out]
                n172 = property on="Test Slider" class="Slide (strict)"("Visible"=FALSE) -> ()  [unwired: 2 in, 2 out]
                n173 = call <vilib>:"NT Read String.vi"("Name"=w302) -> ("String"=w301:string)  [unwired: 9 in, 1 out]
                n174 = Unbundle(w300) -> (w297:string[])
                n175 = Match First String(2:w297, 3:w301) -> (0:w296:i32)  [unwired: 1 out]
                n176 = property on="Test Ring" class="Ring (strict)"("Value"=w296, "Strings []"=w297) -> ()  [unwired: 2 in, 2 out]
              }
              frame "Exposure  **" {
                n177 = Index Array(array=w308, index=2) -> (element=w309:cluster{string[]})
                n178 = property on="Test Ring" class="Ring (strict)"("Visible"=TRUE) -> ()  [unwired: 2 in, 2 out]
                n179 = property on="Test Slider" class="Slide (strict)"("Visible"=FALSE) -> ()  [unwired: 2 in, 2 out]
                n180 = call <vilib>:"NT Read String.vi"("Name"=w311) -> ("String"=w310:string)  [unwired: 9 in, 1 out]
                n181 = Unbundle(w309) -> (w305:string[])
                n182 = Match First String(2:w305, 3:w310) -> (0:w306:i32)  [unwired: 1 out]
                n183 = property on="Test Ring" class="Ring (strict)"("Value"=w306, "Strings []"=w305) -> ()  [unwired: 2 in, 2 out]
              }
              frame "Exposure Priority  **" {
                n184 = Index Array(array=w317, index=3) -> (element=w318:cluster{string[]})
                n185 = property on="Test Ring" class="Ring (strict)"("Visible"=TRUE) -> ()  [unwired: 2 in, 2 out]
                n186 = property on="Test Slider" class="Slide (strict)"("Visible"=FALSE) -> ()  [unwired: 2 in, 2 out]
                n187 = call <vilib>:"NT Read String.vi"("Name"=w320) -> ("String"=w319:string)  [unwired: 9 in, 1 out]
                n188 = Unbundle(w318) -> (w314:string[])
                n189 = Match First String(2:w314, 3:w319) -> (0:w315:i32)  [unwired: 1 out]
                n190 = property on="Test Ring" class="Ring (strict)"("Value"=w315, "Strings []"=w314) -> ()  [unwired: 2 in, 2 out]
              }
              frame "Color Enable  **" {
                n191 = Index Array(array=w326, index=4) -> (element=w327:cluster{string[]})
                n192 = property on="Test Ring" class="Ring (strict)"("Visible"=TRUE) -> ()  [unwired: 2 in, 2 out]
                n193 = property on="Test Slider" class="Slide (strict)"("Visible"=FALSE) -> ()  [unwired: 2 in, 2 out]
                n194 = call <vilib>:"NT Read String.vi"("Name"=w329) -> ("String"=w328:string)  [unwired: 9 in, 1 out]
                n195 = Unbundle(w327) -> (w323:string[])
                n196 = Match First String(2:w323, 3:w328) -> (0:w324:i32)  [unwired: 1 out]
                n197 = property on="Test Ring" class="Ring (strict)"("Value"=w324, "Strings []"=w323) -> ()  [unwired: 2 in, 2 out]
              }
              frame Default {
                n198 = property on="Test Slider" class="Slide (strict)"("Visible"=FALSE) -> ()  [unwired: 2 in, 2 out]
                n199 = property on="Test Ring" class="Ring (strict)"("Visible"=FALSE) -> ()  [unwired: 2 in, 2 out]
              }
              frame "Brightness  **", "Color Level  **", "Compression  **", "FPS  **", "Sharpness  **" {
                n200 = call <vilib>:"NT Read Number.vi"("Name"=w335) -> ("Numeric"=w334:dbl)  [unwired: 9 in, 1 out]
                n201 = property on="Test Ring" class="Ring (strict)"("Visible"=FALSE) -> ()  [unwired: 2 in, 2 out]
                n202 = property on="Test Slider" class="Slide (strict)"("Visible"=TRUE, "Scale.Maximum"=100.0 ("Scale.Range:Maximum")) -> ()  [unwired: 2 in, 2 out]
                n203 = local write "Test Slider"(w334) -> ()
              }
            }
            n204 = property on="Motor" class="Clust (strict)"("Visible"=FALSE) -> ()  [unwired: 2 in, 2 out]
          }
        }
      }
      event "Test Name": Mouse Enter {
        # "Populate the ring with the list of tests"
        n205 = event-data() -> ()  [unwired: 1 in, 1 out]
        n206 = call <vilib>:"NT Read String Array.vi"("Name"="TestMode/TestList") -> ("String Array"=w343:string[])  [unwired: 9 in, 1 out]
        n207 = Build Array (concatenate)("Select the test to run...", w343) -> (w342:string[])
        n208 = property on="Test Name" class="Ring (strict)"("Strings []"=w342) -> ()  [unwired: 2 in, 2 out]
      }
      event "Test Name": Value Change {
        w345 = FALSE ("Visible")
        # "Tell the robot the test name to run"
        n209 = event-data() -> ("NewVal"=w349:u16)  [unwired: 1 in]
        n210 = property on="Test Name" class="Ring (strict)"() -> ("Strings []"=w350:string[])  [unwired: 2 in, 2 out]
        n211 = local write "Progress"(T8 {"Test Progress"=0, "Test Progress Text"=""} ("Progress")) -> ()
        n212 = property on="Test Ring" class="Ring (strict)"("Visible"=w345) -> ()  [unwired: 2 in, 2 out]
        n213 = property on="Motor" class="Clust (strict)"("Visible"=w345) -> ()  [unwired: 2 in, 2 out]
        n214 = property on="Test Slider" class="Slide (strict)"("Visible"=w345) -> ()  [unwired: 2 in, 2 out]
        n215 = property on="On/Off" class="Bool (strict)"("Visible"=w345) -> ()  [unwired: 2 in, 2 out]
        n216 = property on="Rev/Fwd" class="Clust (strict)"("Visible"=w345) -> ()  [unwired: 2 in, 2 out]
        n217 = property on="Progress" class="Clust (strict)"("Visible"=TRUE) -> ()  [unwired: 2 in, 2 out]
        n218 = Index Array(array=w350, index=w349) -> (element=w348:string)
        n219 = call <vilib>:"NT Write String.vi"("String"=w348, "Name"="TestMode/TestName") -> ()  [unwired: 9 in, 1 out]
      }
      event "Listbox": Double Click {
        n220 = event-data() -> ("PlatMods.Shift"=w353:bool, "Row"=w355:i32)  [unwired: 1 in]
        n221 = case shown="True" w353 {
          tunnel: w355 -> [w359 _]
          tunnel: 1 -> [w358 _]
          frame False {
            n222 = property on="Listbox" class="LstBox (strict)"() -> ("Item Symbols"=w357:i32[])  [unwired: 2 in, 2 out]
            n223 = Replace Array Subset(array=w357, new element=w358, index=w359) -> (w356:i32[])
            n224 = property on="Listbox" class="LstBox (strict)"("Item Symbols"=w356) -> ()  [unwired: 2 in, 2 out]
          }
          frame True {
            w360 = 0 ("Top Row")
            n225 = property on="Listbox" class="LstBox (strict)"() -> ("Number of Rows"=w362:u32)  [unwired: 2 in, 2 out]
            n226 = Initialize Array(0, w362) -> (w361:i32[])
            n227 = property on="Listbox" class="LstBox (strict)"("Top Row"=w360, "Value"=w360, "Item Symbols"=w361) -> ()  [unwired: 2 in, 2 out]
          }
        }
      }
      event "Listbox": Key Down {
        n228 = event-data() -> ("VKey"=w366:T17)  [unwired: 1 in]
        n229 = case shown="\"Left\", \"Right\"" w366 {
          selector: w366 -> [w371 _]
          tunnel: eventvkey."Left" ("VKey") -> [w369 _]
          frame "Left", "Right" {
            n230 = Equal?(x=w369, y=w371) -> (x = y?=w370:bool)
            n231 = Select(t=0, s=w370, f=1) -> (s? t:f=w372:i32)
            n232 = property on="Listbox" class="LstBox (strict)"() -> ("Item Symbols"=w375:i32[])  [unwired: 2 in, 2 out]
            n233 = Replace Array Subset(array=w375, new element=w372, index="Listbox") -> (w374:i32[])
            n234 = property on="Listbox" class="LstBox (strict)"("Item Symbols"=w374) -> ()  [unwired: 2 in, 2 out]
          }
          frame Default {
          }
        }
      }
      event "DB Camera Config": Value Change {
        n235 = event-data() -> ("NewVal"=w379:bool)  [unwired: 1 in]
        n236 = case shown="False" w379 {
          tunnel: w378 -> [w388 _]
          tunnel: [w381 w399] -> w377
          tunnel: w376 -> [w380 w399]
          frame False {
            w395 = "Camera"
            w398 = FALSE ("Visible")
            n237 = property on="Camera Settings" class="Clust (strict)"("Visible"=w398) -> ()  [unwired: 2 in, 2 out]
            n238 = local write "DB Camera Config"(w398) -> ()
            n239 = local read "Camera Settings"() -> (w387:T3)
            n240 = Index Array(array=w388) -> (element=w391:cluster{string[]})  [unwired: 1 in]
            n241 = Unbundle(w391) -> (w390:string[])
            n242 = Unbundle(w387) -> ("Frame Rate"=w386:i32, "Compression"=w385:i32, "Size"=w389:u16)
            n243 = Index Array(array=w390, index=w389) -> (element=w384:string)
            n244 = call-poly <vilib>:"Write Key.vi"("section"=w395, "value"=w384, "key"="Size", "refnum"=w380) -> ("refnum out"=w397:T13)  [unwired: 2 in, 5 out]
            n245 = call-poly <vilib>:"Write Key.vi"("section"=w395, "value"=w386, "key"="FrameRate", "refnum"=w397) -> ("refnum out"=w396:T13)  [unwired: 1 in, 6 out]
            n246 = call-poly <vilib>:"Write Key.vi"("section"=w395, "value"=w385, "key"="Compression", "refnum"=w396) -> ("refnum out"=w382:T13)  [unwired: 1 in, 6 out]
            n247 = call <vilib>:"Close Config Data.vi"("refnum"=w382) -> ("file path"=w383:path)  [unwired: 2 in, 8 out]
            n248 = call <vilib>:"Open Config Data.vi"("configuration file path"=w383) -> ("refnum"=w381:T13)  [unwired: 8 in, 2 out]
          }
          frame True {
            n249 = property on="Camera Settings" class="Clust (strict)"("Visible"=TRUE) -> ()  [unwired: 2 in, 2 out]
          }
        }
      }
      event "Camera Settings": Value Change {
        n250 = event-data() -> ("NewVal"=w412:T3)  [unwired: 1 in]
        n251 = Index Array(array=w408) -> (element=w407:cluster{string[]})  [unwired: 1 in]
        n252 = Unbundle(w412) -> ("Frame Rate"=w403:i32, "Compression"=w402:i32, "Size"=w405:u16)
        n253 = Unbundle(w407) -> (w406:string[])
        n254 = Index Array(array=w406, index=w405) -> (element=w404:string)
        n255 = Format Into String(format string="%s   %dfps   %d%%", w404, w403, w402) -> (resulting string=w409:string)  [unwired: 2 in, 1 out]
        n256 = Build Array(w409) -> (w410:string[])
        n257 = property on="DB Camera Config" class="Bool (strict)"("Strings [4]"=w410) -> ()  [unwired: 2 in, 2 out]
      }
      event "Motor.Enable": Value Change {
        n258 = event-data() -> ("NewVal"=w418:bool)  [unwired: 1 in]
        n259 = Unbundle("Motor") -> ("Value"=w417:dbl)  [unwired: 1 out]
        n260 = Select(t=w417, s=w418, f=0.0) -> (s? t:f=w415:dbl)
        n261 = call <vilib>:"NT Write Number.vi"("Numeric"=w415, "Name"=w414) -> ()  [unwired: 9 in, 1 out]
      }
      event "Test Slider": Value Change {
        n262 = event-data() -> ("NewVal"=w421:dbl)  [unwired: 1 in]
        n263 = call <vilib>:"NT Write Number.vi"("Numeric"=w421, "Name"=w422) -> ()  [unwired: 9 in, 1 out]
      }
      event "On/Off": Value Change {
        n264 = event-data() -> ("NewVal"=w426:bool)  [unwired: 1 in]
        n265 = Boolean To (0,1)(Boolean=w426) -> (0, 1=w425:i16)
        n266 = call <vilib>:"NT Write Number.vi"("Numeric"=w425, "Name"=w424) -> ()  [unwired: 9 in, 1 out]
      }
      event "Rev/Fwd": Value Change {
        n267 = event-data() -> ("NewVal.Forward"=w434:bool, "NewVal.Reverse"=w433:bool)  [unwired: 1 in]
        n268 = Boolean To (0,1)(Boolean=w433) -> (0, 1=w432:i16)
        n269 = Boolean To (0,1)(Boolean=w434) -> (0, 1=w430:i16)
        n270 = Negate(x=w432) -> (-x=w431:i16)
        n271 = Add(x=w430, y=w431) -> (x+y=w429:i16)
        n272 = call <vilib>:"NT Write Number.vi"("Numeric"=w429, "Name"=w428) -> ()  [unwired: 9 in, 1 out]
      }
      event "Test Ring": Value Change {
        n273 = event-data() -> ("NewVal"=w438:u16)  [unwired: 1 in]
        n274 = property on="Test Ring" class="Ring (strict)"() -> ("Strings []"=w439:string[])  [unwired: 2 in, 2 out]
        n275 = Index Array(array=w439, index=w438) -> (element=w437:string)
        n276 = call <vilib>:"NT Write String.vi"("String"=w437, "Name"=w436) -> ()  [unwired: 9 in, 1 out]
      }
      event "Rec Mode": Value Change {
        # "Update globals for recording mode and path to read log from.\nClear when logging and let NetworkTables set path for vision to\nuse."
        n277 = event-data() -> ("NewVal"=w447:enum32{"Stop", "Record", "Playback"})  [unwired: 1 in]
        n278 = global write "WPI_DashboardLogging Global.vi" "Logging Filename"(path "") -> ()
        n279 = call <vilib>:"WPI_DashboardNT Log FieldName Cache.vi"("Operation"=enum16{"Lookup/Add", "Index", "Clear"}."Clear") -> ()  [unwired: 8 in, 3 out]
        n280 = global write "WPI_DashboardLogging Global.vi" "Recording"(w447) -> ()
        n281 = case shown="\"Stop\", \"Record\"" w447 {
          tunnel: w446 -> [_ w449 w457]
          tunnel: [_ _ w456] -> w443
          tunnel: [_ _ w455] -> _
          tunnel: w441 -> [_ _ w453]
          tunnel: cluster{i32, i32} {-250, 170} -> [_ _ w452]
          tunnel: [_ _ T18 {"Image Size"=TRUE, "Image Type"=TRUE, "Pixel Value"=TRUE, "ROI Information"=TRUE, "Zoom Factor"=FALSE} ("Image Information Shown:All Elements")] -> _
          tunnel: [_ _ TRUE ("Zoom Factor")] -> _
          frame Default {
          }
          frame "Stop", "Record" {
            # "Place Window too"
            n282 = invoke class="VI" method="FP.Close"(reference=w449) -> (reference out=w448:refnum<vi>)  [unwired: 2 in, 2 out]
            n283 = invoke class="VI" method="Abort VI"(reference=w448) -> ()  [unwired: 2 in, 3 out]
          }
          frame "Playback" {
            n284 = call "Open Playback Panel.vi"("Offset"=w452, "DB VI Ref"=w453, "Playback in"=w457) -> ("Playback out"=w454:refnum<vi>)  [unwired: 8 in]
            n285 = register-events(w454) -> (reference out=w456:refnum<event-registration>, error out=w455:errorcluster)  [unwired: 2 in]
          }
        }
      }
      event Panel Close {
        w458 = enum32{"Stop", "Record", "Playback"}."Stop" ("Rec Mode")
        n286 = event-data() -> ()  [unwired: 1 in, 4 out]
        n287 = local write "Rec Mode"(w458) -> ()
        n288 = global write "WPI_DashboardLogging Global.vi" "Recording"(w458) -> ()
      }
      event Panel Close {
        # "Abort playback window and ourself"
        n289 = event-data() -> ()  [unwired: 1 in, 4 out]
        n290 = invoke class="VI" method="FP.Close"(reference=w463) -> (reference out=w462:refnum<vi>)  [unwired: 2 in, 2 out]
        n291 = invoke class="VI" method="Abort VI"(reference=w462) -> (error out=w461:errorcluster)  [unwired: 2 in, 2 out]
        n292 = invoke class="VI" method="Abort VI"(error in=w461) -> ()  [unwired: 2 in, 3 out]
      }
    }
  }
